vi "example -01- simple commands.vi"() -> ()   [LabVIEW 2019, in "mmW_commands.lvlib"]
uses:
  mmW_commands.lvlib
  TypeDefs/commands.ctl
  commands/configure_rf.ctl
  e0d3282b-1062-443e-8354-34e5993a984c.vi
  177f26ca-89ca-4335-9970-cb64af06c064.vi
  commands/_depr_initialize_hw.ctl
  dcd0e113-c981-49df-98fb-02ece35e15ae.vi
  commands/shutdown_typedef.ctl
  fb3c95a4-d458-4604-b9e0-1c3e2e2b5bec.vi
panel:
  out "type out 3":T1
  out "type out 2":T1
  out "initialize hw":T2
  out "type out":T3
  out "Test case":T4=enum."configure_rf"
  in  "Run":bool
  out "error out":errorcluster
  out "Debug info":string
  out "Valid message?":bool
  out "command out":T4=enum."configure_rf"
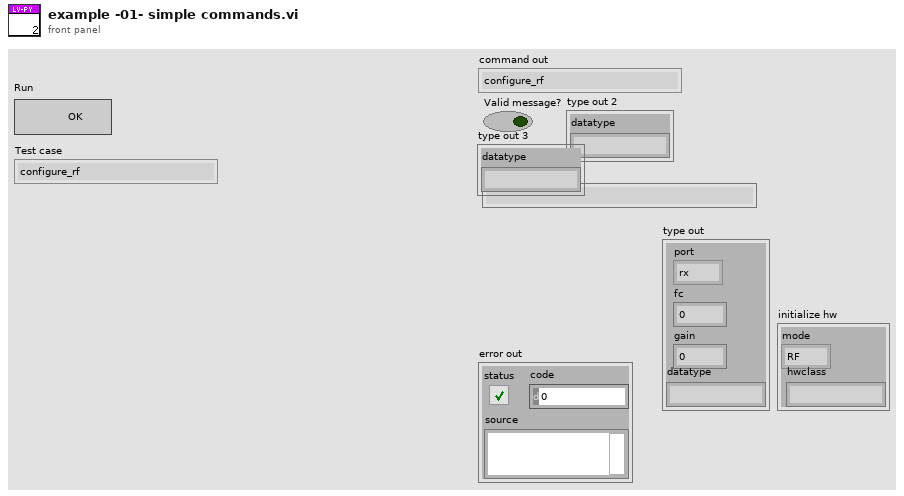
[diagram p1: front panel]
types:
  T1 = typedef "mmW_commands.lvlib/shutdown_typedef.ctl" = cluster{"datatype":string}
  T2 = typedef "mmW_commands.lvlib/_depr_initialize_hw.ctl" = cluster{"mode":enum16{"RF", "IF", "BB"}, "hwclass":string}
  T3 = typedef "mmW_commands.lvlib/configure_rf.ctl" = cluster{"port":enum16{"rx", "tx"}, "fc":dbl, "gain":dbl, "datatype":string}
  T4 = typedef "mmW_commands.lvlib/commands.ctl" = enum16{"configure_fs", "configure_rf", "configure_trigger", "equalization_enable", "equalization_start", "lo_sync_enable", "equalization_stop", "get_instrument_status", "get_versions", "initialize_hw", "pop_rx", "set_log_level", "Shutdown", "start", "start_instrument_app", "stop", "trans", "transceive", "trigger_burst", "trigger_sync_enable", "Write TX", "resp_generic", "resp_waveform", "send_trigger", "fetch", "transceive2"}
  T5 = typedef "mmW_commands.lvlib/commands_instrument_control.ctl" = enum16{"configure_rf", "configure_rx_sync", "configure_trigger", "initialize_hw", "pop_rx", "set_mode", "shutdown", "start", "stop", "trigger_burst", "write_tx", "transceive"}
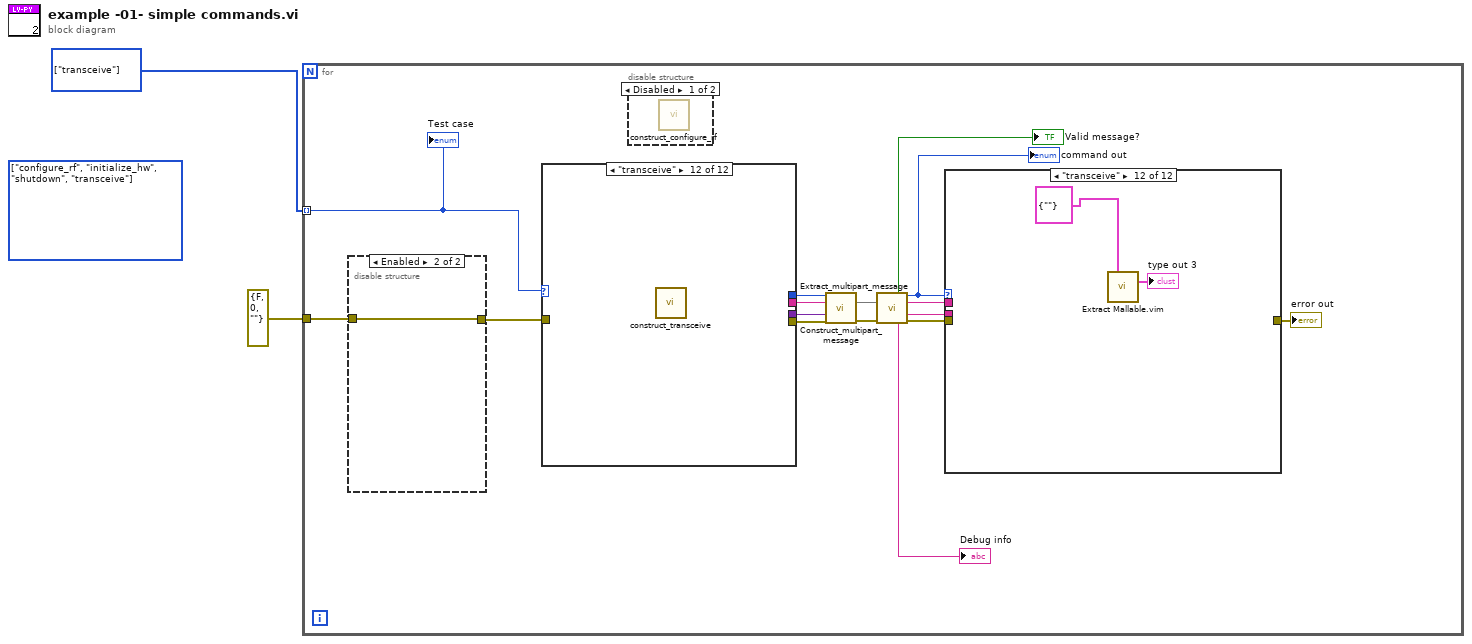
[diagram p0: block diagram]
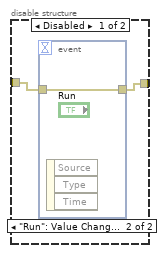
[diagram p3: hidden frame]
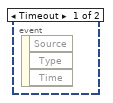
[diagram p4: hidden frame]
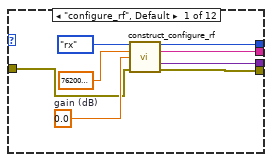
[diagram p5: hidden frame]
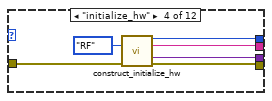
[diagram p8: hidden frame]
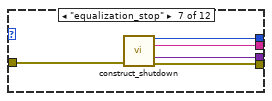
[diagram p11: hidden frame]
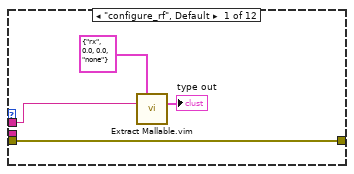
[diagram p16: hidden frame]
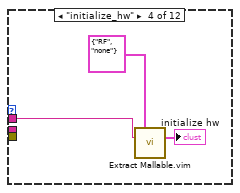
[diagram p19: hidden frame]
diagram:
  w1 = T4[] [enum."transceive"] items=["configure_fs", "configure_rf", "configure_trigger", "equalization_enable", "equalization_start", "lo_sync_enable", "equalization_stop", "get_instrument_status", "get_versions", "initialize_hw", "pop_rx", "set_log_level", "Shutdown", "start", "start_instrument_app", "stop", "trans", "transceive", "trigger_burst", "trigger_sync_enable", "Write TX", "resp_generic", "resp_waveform", "send_trigger", "fetch", "transceive2"]
  (unwired) T5[] [enum."configure_rf", enum."initialize_hw", enum."shutdown", enum."transceive"] items=["configure_rf", "configure_rx_sync", "configure_trigger", "initialize_hw", "pop_rx", "set_mode", "shutdown", "start", "stop", "trigger_burst", "write_tx", "transceive"]
  n1 = for {
    tunnel: w1 -> [w15] mode=indexing
    tunnel: errorcluster {"status"=FALSE, "code"=0, "source"=""} ("error out") -> [w4]
    n2 = disable-structure shown="Enabled" {
      disable-tunnel: w4 -> [w20 w22]
      disable-tunnel: [w19 w22] -> w3
      frame Disabled {
        n3 = event shown="[1] \"Run\": Value Change" {
          selector: _ -> [_ _]
          dyn-events: _ -> [_ _]
          timeout: _ -> [_ _]
          tunnel: w20 -> [_ w21]
          tunnel: [_ w21] -> w19
          event Timeout {
            n4 = event-data() -> ()  [unwired: 1 in, 3 out]
          }
          event "Run": Value Change {
            n5 = event-data() -> ()  [unwired: 1 in, 3 out]
          }
        }
      }
      frame Enabled {
      }
    }
    n6 = case shown="\"transceive\"" w15 {
      tunnel: [w27 _ _ w36 _ _ w41 _ _ _ _ _] -> w12
      tunnel: [w26 _ _ w35 _ _ w40 _ _ _ _ _] -> w11
      tunnel: [w25 _ _ w34 _ _ w39 _ _ _ _ _] -> w10
      tunnel: [w24 _ _ w33 _ _ w38 _ _ _ _ _] -> w9
      tunnel: w3 -> [w23 _ _ w32 _ _ w37 _ _ _ _ _]
      frame "configure_rf", Default {
        w28 = 0.0  # gain (dB)
        n7 = call "construct_configure_rf.vi"("port"=enum16{"rx", "tx"}."rx", "fc (Hz)"=76200000000.0, "gain (dB)"=w28, "error in (no error)"=w23) -> ("command out"=w27:T4, "parameters JSON"=w26:string, "data out"=w25:variant, "error out"=w24:errorcluster)  [unwired: 7 in, 1 out]
      }
      frame "configure_rf" {
      }
      frame "configure_trigger" {
      }
      frame "initialize_hw" {
        n8 = call "construct_initialize_hw.vi"("Mode"=enum16{"RF", "IF", "BB"}."RF", "error in (no error) 2"=w32) -> ("command out"=w36:T4, "parameters JSON"=w35:string, "data out"=w34:variant, "error out 2"=w33:errorcluster)  [unwired: 9 in, 1 out]
      }
      frame "pop_rx" {
      }
      frame "lo_sync_enable" {
      }
      frame "equalization_stop" {
        n9 = call "construct_shutdown.vi"("error in (no error) 2"=w37) -> ("command out"=w41:T4, "parameters JSON"=w40:string, "data out"=w39:variant, "error out 2"=w38:errorcluster)  [unwired: 10 in, 1 out]
      }
      frame "start" {
      }
      frame "stop" {
      }
      frame "trigger_burst" {
      }
      frame "Shutdown" {
      }
      frame "transceive" {
        n10 = call "construct_transceive.vi"() -> ()  [unwired: 11 in, 5 out]
      }
    }
    n11 = disable-structure shown="Disabled" {
      frame Disabled {
        n12 = call "construct_configure_rf.vi"() -> ()  [unwired: 11 in, 5 out]
      }
      frame Enabled {
      }
    }
    n13 = call "Construct_multipart_message.vi"("command"=w12, "parameters (JSON)"=w11, "data in"=w10, "error in (no error)"=w9) -> (6:w18, "error out"=w17:errorcluster)  [unwired: 7 in, 3 out]
    n14 = call "Extract_multipart_message.vi"(5:w18, "error in (no error)"=w17) -> ("Valid message?"=→"Valid message?":bool, "command out"=w16:T4, "parameters"=w14:string, "data out"=w13:string, "Debug info"=→"Debug info":string, "error out"=w6:errorcluster)  [unwired: 6 in, 2 out]
    "command out" <- w16
    n15 = case shown="\"transceive\"" w16 {
      tunnel: w14 -> [w43 _ _ w47 _ _ w51 _ _ _ _ _]
      tunnel: w13 -> [_ _ _ _ _ _ _ _ _ _ _ _]
      tunnel: w6 -> [w45 _ _ _ _ _ _ _ _ _ _ _]
      tunnel: [w45 _ _ _ _ _ _ _ _ _ _ _] -> w5
      frame "configure_rf", Default {
        n16 = call "Extract Mallable.vim"("type in"=T3 {"port"=enum."rx", "fc"=0.0, "gain"=0.0, "datatype"="none"} ("Cluster"), "JSON in"=w43) -> ("type out"=→"type out":T3)  [unwired: 13 in]
      }
      frame "configure_rf" {
      }
      frame "configure_trigger" {
      }
      frame "initialize_hw" {
        n17 = call "Extract Mallable.vim"("type in"=T2 {"mode"=enum."RF", "hwclass"="none"} ("Cluster"), "JSON in"=w47) -> ("type out"=→"initialize hw":T2)  [unwired: 13 in]
      }
      frame "pop_rx" {
      }
      frame "lo_sync_enable" {
      }
      frame "equalization_stop" {
        n18 = call "Extract Mallable.vim"("type in"=T1 {"datatype"=""} ("Cluster"), "JSON in"=w51) -> ("type out"=→"type out 2":T1)  [unwired: 13 in]
      }
      frame "start" {
      }
      frame "stop" {
      }
      frame "trigger_burst" {
      }
      frame "Shutdown" {
      }
      frame "transceive" {
        n19 = call "Extract Mallable.vim"("type in"=T1 {"datatype"=""} ("Cluster")) -> ("JSON in"=w54:string, "type out"=→"type out 3":T1)  [unwired: 13 in]
      }
    }
    "error out" <- w5
    "Test case" <- w15
  }
